vi "Read Rooms.vi"(8 "error in (no error)":errorcluster, 11 "Door":refnum<class "Door.lvclass">) -> (0 "error out":errorcluster, 2 "Rooms":refnum<class "Room.lvclass">[](array[class]), 3 "Door":refnum<class "Door.lvclass">)   [LabVIEW 2020, in "Door.lvclass"]
uses:
  Door.lvclass
  Room/Room.lvclass
  Door.lvclass/Door.ctl
  Private/TypeDef/privateDataDVR.ctl
  Private/TypeDef/privateData.ctl
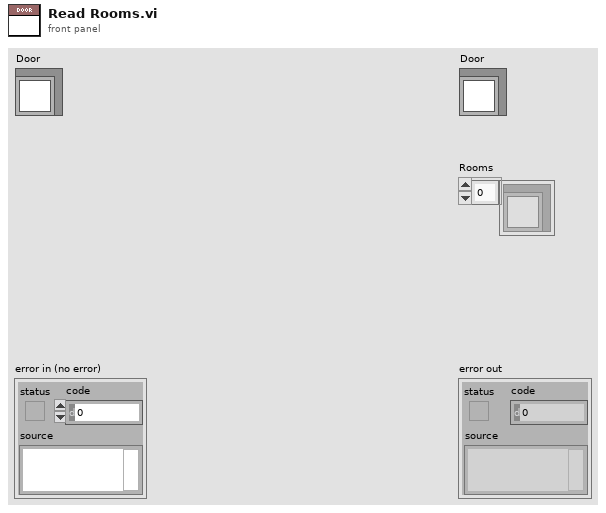
[diagram p1: front panel]
types:
  T1 = typedef "Door.lvclass/privateDataDVR.ctl" = refnum<data-value>
  T2 = typedef "Door.lvclass/privateData.ctl" = cluster{"room1":refnum<class "Room.lvclass">, "room2":refnum<class "Room.lvclass">}
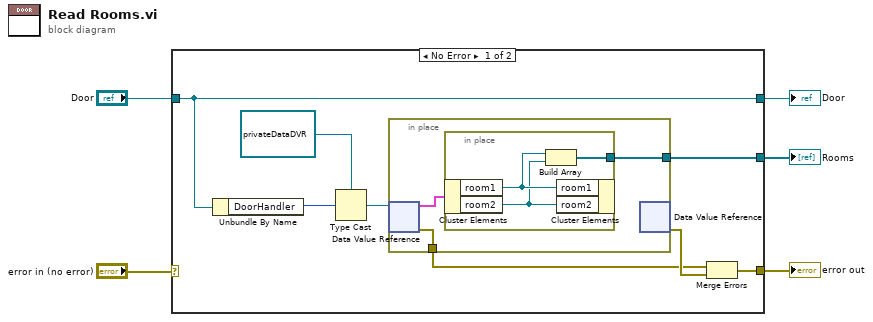
[diagram p0: block diagram]
diagram:
  n1 = case shown="No Error" "error in (no error)" {
    selector: "error in (no error)" -> [_ w20]
    tunnel: "Door" -> [w9 w21]
    tunnel: [w9 w21] -> w4
    tunnel: [w8 w20] -> w3
    tunnel: [w6 _] -> w1
    frame No Error {
      n2 = Unbundle By Name(w9) -> ("DoorHandler"=w11:u32)
      n3 = Type Cast(type=T1 refnum ("privateDataDVR"), x=w11) -> (*(type *) &x=w13:T1)
      n4 = in-place {
        in-place-border: [w15] -> w10
        in-place-border: [w14] -> w6
        n5 = in-place-dvr #1(w13) -> (w16:T2, w15:errorcluster)
        n6 = in-place {
          in-place-border: [w17] -> w14
          n7 = in-place-cluster #2(w16) -> ("room1"=w19:refnum<class "Room.lvclass">, "room2"=w18:refnum<class "Room.lvclass">)
          n8 = Build Array(w19, w18) -> (w17:refnum<class "Room.lvclass">[])
          n9 = in-place-cluster #2("room1"=w19, "room2"=w18) -> ()  [unwired: 1 out]
        }
        n10 = in-place-dvr #1() -> (w12:errorcluster)  [unwired: 1 in, 1 out]
      }
      n11 = Merge Errors(w10, w12) -> (w8:errorcluster)
    }
    frame Error {
    }
  }
  "error out" <- w3
  "Door" <- w4
  "Rooms" <- w1
